vi "doAction.vi"(8 "error in (no error)":errorcluster, 10 "ContextData.lvclass":refnum<class "ContextData.lvclass">, 11 "Wait Event in":refnum<class "Wait Event.lvclass">) -> (0 "error out":errorcluster, 3 "Wait Event out":refnum<class "Wait Event.lvclass">)   [LabVIEW 2018, in "Wait Event.lvclass"]
uses:
  Wait Event.lvclass
  ContextData/ContextData.lvclass
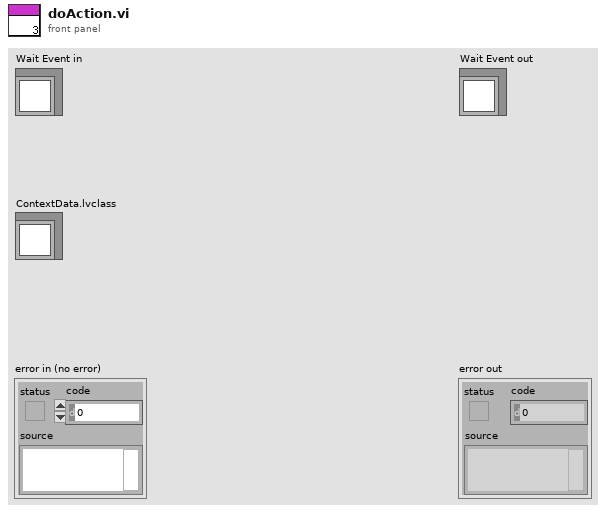
[diagram p1: front panel]
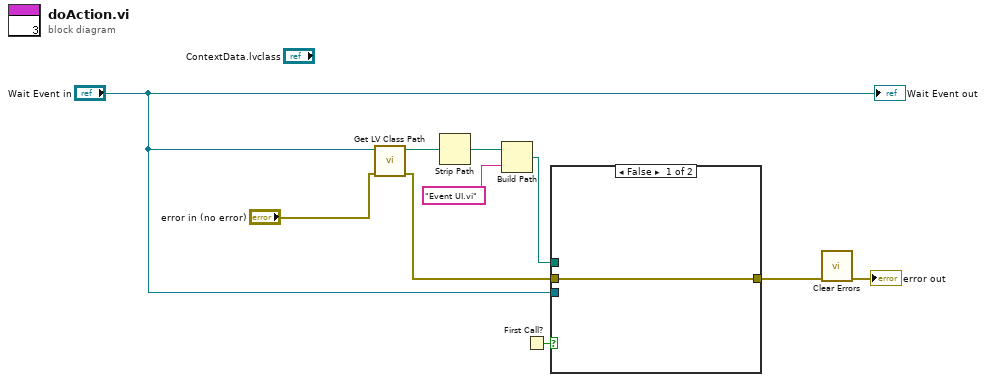
[diagram p0: block diagram]
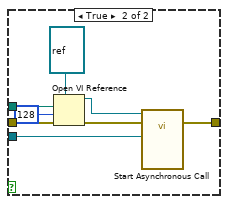
[diagram p2: hidden frame]
diagram:
  n1 = call <vilib>:"Get LV Class Path.vi"("error in (no error)"="error in (no error)", "object"="Wait Event in") -> ("error out"=w8:errorcluster, "class path"=w10:path)  [unwired: 8 in]
  n2 = Strip Path(path=w10) -> (stripped path=w5:path)  [unwired: 1 out]
  n3 = Build Path(base path=w5, name or relative path="Event UI.vi") -> (appended path=w6:path)
  n4 = First Call?() -> (First Call?: T/F=w1:bool)
  n5 = case shown="False" w1 {
    tunnel: w8 -> [w11 w19]
    tunnel: w6 -> [_ w18]
    tunnel: "Wait Event in" -> [_ w17]
    tunnel: [w11 w14] -> w2
    frame False {
    }
    frame True {
      n6 = Open VI Reference(type specifier VI Refnum (for type only)=refnum<vi> refnum, vi path=w18, options=128, error in (no error)=w19) -> (vi reference=w13:refnum<vi>, error out=w16:errorcluster)  [unwired: 2 in]
      n7 = call-by-ref "Start Asynchronous Call"(reference=w13, error in=w16, "Wait Event in"=w17) -> (error out=w14:errorcluster)  [unwired: 9 in, 3 out]
    }
  }
  n8 = call <vilib>:"Clear Errors.vi"("error in (no error)"=w2) -> ("error out"=→"error out":errorcluster)  [unwired: 5 in, 1 out]
  "Wait Event out" <- "Wait Event in"
